vi "Drive Controller.vi"(8 "error in":errorcluster) -> ()   [LabVIEW 2018]
doc: "This VI executes continuously carrying out the current operation and responding to updates or new operation requests. It will often contain the timing or control code that is difficult to place directly in TeleOp. This VI generally opens all sensors and motors and isolates the rest of the robot code from knowing implementation details of how the operations are carried out."
uses:
  <vilib>/Rock Robotics/WPI/Framework/Completion Status.ctl
  2018 Practice Mecanum Command and Control/Drive/Implementation/Drive Setpoints.ctl
  2018 Practice Mecanum Command and Control/Drive/Implementation/Drive Operations.ctl
  <vilib>/Rock Robotics/WPI/SafetyOutput/WPI_SafetyOutputConfigMenu.ctl
  <vilib>/Rock Robotics/WPI/RobotDrive/WPI_RobotDriveOpen2MotorWithTalon.vi
panel:
  in  "Interactive Values":T1
  in  "Buttons":cluster{"Execute Cmd":bool, "Abort Cmd":bool}
  out "Command Timing":cluster{"Start Time (ms)":u32, "Iterations":i32}
  out "Status":T3
  out "Setpoints":T4(graph)
  out "Current\nCmd":string
  # "Tip: The graph shows the motor setpoints. It may also be helpful to observe inputs and sensor values.\nYou may also want to display tuning or debugging controls."
  # "Interactive Command: You may fill in the settings for a command\nand schedule it with the Execute button. You can observe and abort\nany command while fine tuning the code for the controller."
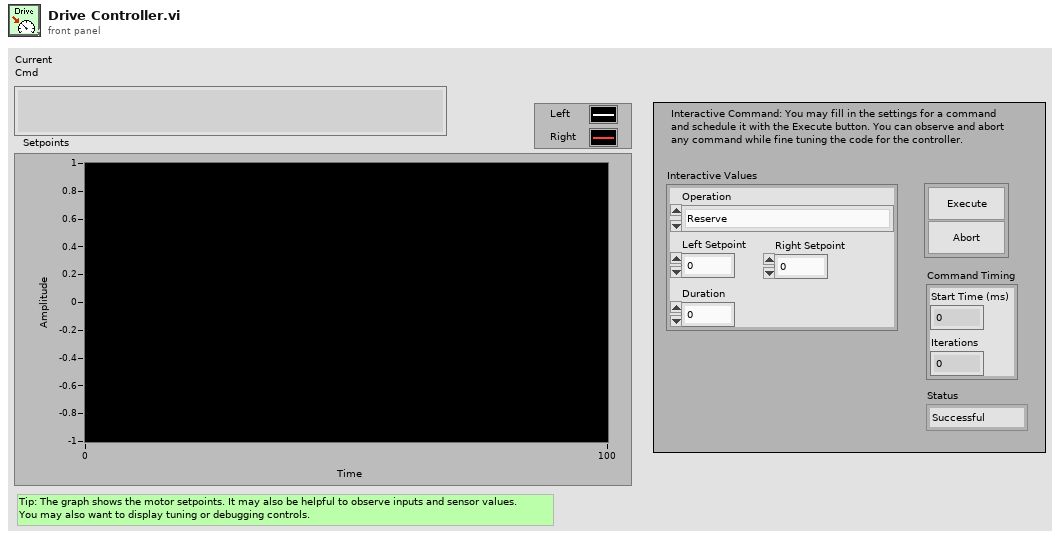
[diagram p1: front panel]
types:
  T1 = typedef "Drive Setpoints.ctl" = cluster{"Operation":T2, "Left Setpoint":dbl, "Right Setpoint":dbl, "Duration":dbl}
  T2 = typedef "Drive Operations.ctl" = enum16{"Reserve", "Read Current", "Immediate", "Drive for Time", "Drive for Distance"}
  T3 = typedef "Completion Status.ctl" = enum16{"Successful", "Aborted", "Incomplete"}
  T4 = cluster{"Left Setpoint":dbl, "Right Setpoint":dbl}
  T5 = typedef "WPI_SafetyOutputConfigMenu.ctl" = enum16{"Enable", "Disable"}
  T6 = typedef "WPI_RobotDriveDevRef.ctl" = cluster{"DevStatus":errorcluster, "Motors[]":T7[], "Square Inputs":bool, "Max Output":dbl}
  T7 = typedef "WPI_MotorControlDeviceRef.ctl" = cluster{"DeviceStatus":errorcluster, "Type":T8, "PWM":cluster{"PWM Channel":T9, "DeadBand":T10}, "CAN":cluster{"Device Number":u8, "SetOutput VI Ref":variant, "GetOutput VI Ref":variant, "Enable VI Ref":variant, "Disable VI Ref":variant, "Data":variant}, "Invert":bool, "DIO PWM":cluster{"PWM \"Enable\" Channel":T9, "DIOChannel":T11, "PWM Rate":dbl}}
  T8 = typedef "WPI_MotorControlType.ctl" = enum16{"PWM", "CAN", "DIO PWM"}
  T9 = typedef "FPGA_DIOPWMChannel.ctl" = enum8{"PWM 0", "PWM 1", "PWM 2", "PWM 3", "PWM 4", "PWM 5", "PWM 6", "PWM 7", "PWM 8", "PWM 9", "PWM MXP 0", "PWM MXP 1", "PWM MXP 2", "PWM MXP 3", "PWM MXP 4", "PWM MXP 5", "PWM MXP 6", "PWM MXP 7", "PWM MXP 8", "PWM MXP 9", "Invalid"}
  T10 = typedef "WPI_PWMDeadband.ctl" = cluster{"Name":string, "maxPositivePwm":i32, "minPositivePwm":i32, "centerPwm":i32, "maxNegativePwm":i32, "minNegativePwm":i32, "angularRange":u16}
  T11 = typedef "FPGA_DIOChannel.ctl" = enum8{"DIO 0", "DIO 1", "DIO 2", "DIO 3", "DIO 4", "DIO 5", "DIO 6", "DIO 7", "DIO 8", "DIO 9", "DIO MXP 0", "DIO MXP 1", "DIO MXP 2", "DIO MXP 3", "DIO MXP 4", "DIO MXP 5", "DIO MXP 6", "DIO MXP 7", "DIO MXP 8", "DIO MXP 9", "DIO MXP 10", "DIO MXP 11", "DIO MXP 12", "DIO MXP 13", "DIO MXP 14", "DIO MXP 15", "SPI Port CS1", "SPI Port CS2", "SPI Port CS3", "SPI Port MISO", "SPI Port MOSI", "Invalid"}
  T12 = typedef "Command Status Info.ctl" = cluster{"Name":string, "Status":T3, "notifier out":T13}
  T13 = typedef "Completion Notifier.ctl" = refnum<notifier>
  T14 = cluster{"SubSystem Data":T1, cluster{"Start Time (ms)":u32, "Iterations":i32}, cluster{"Command Info":T12, "Description":string, "Default Command":T1, "queue out":refnum<queue>, "Subsystem Name":string}}
  T15 = cluster{"SubSystem Data":T1, cluster{"Start Time (ms)":u32, "Iterations":i32}, "Default Command Arguments":cluster{"Command Info":T12, "Description":string, "Default Command":T1, "queue out":refnum<queue>, "Subsystem Name":string}}
  T16 = cluster{"Don't move motors while reserved":dbl, "Don't move motors while reserved":dbl}
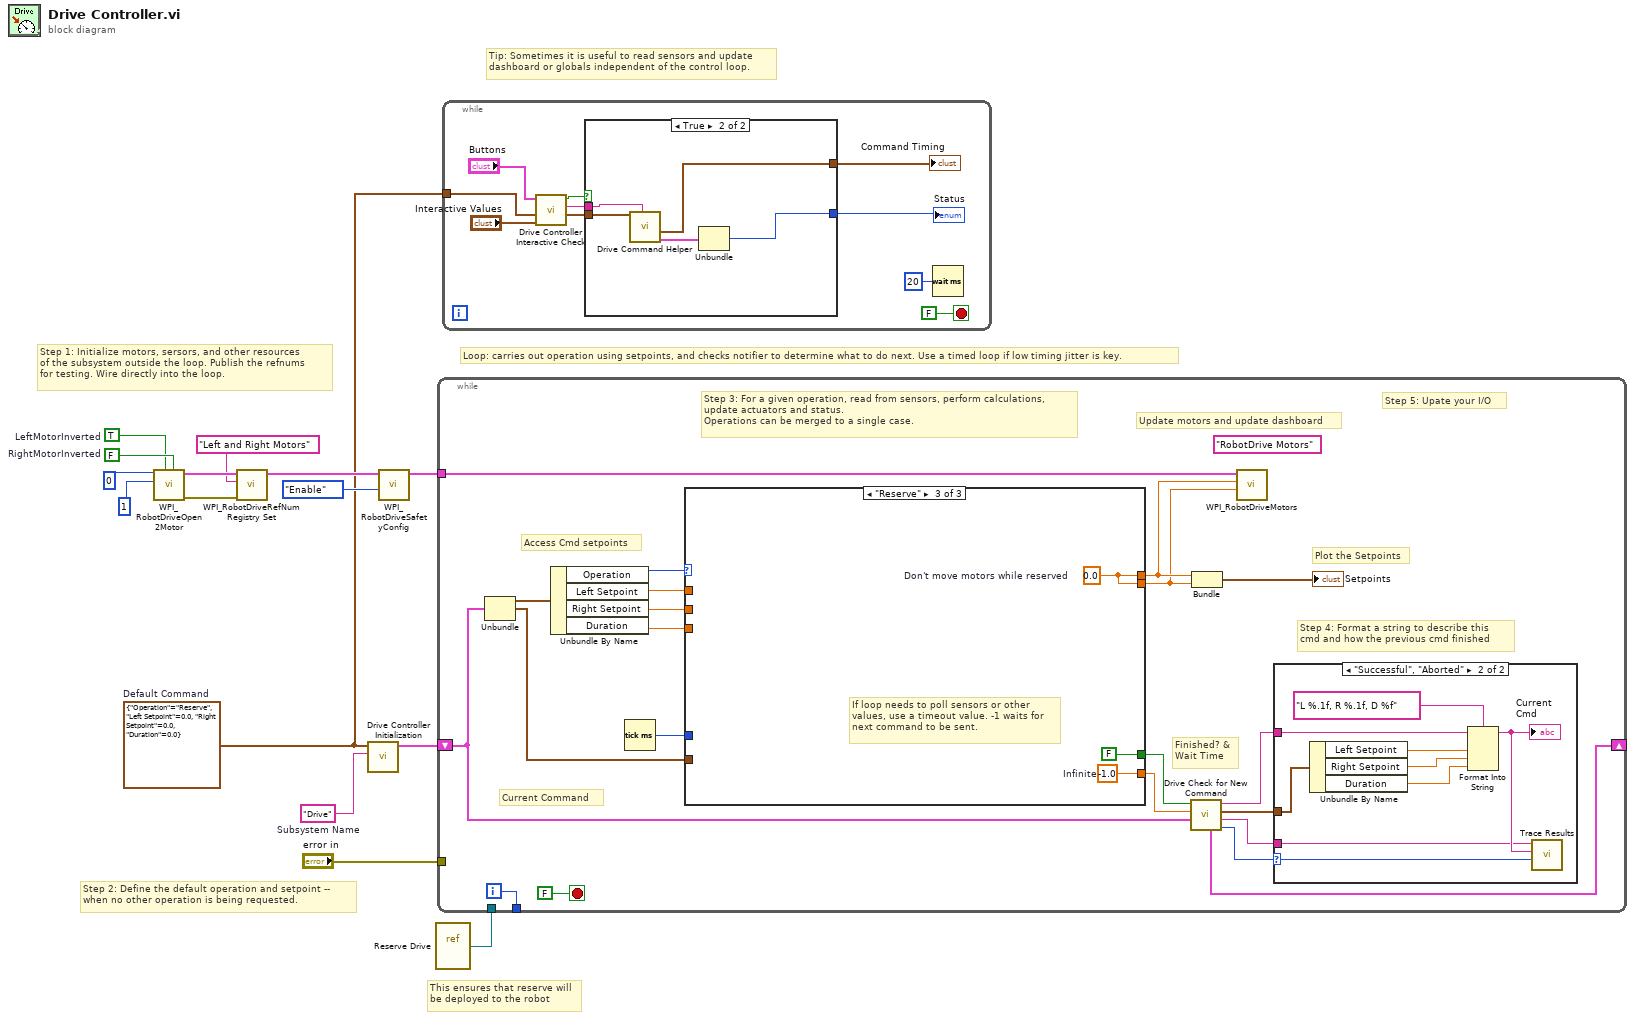
[diagram p0: block diagram]
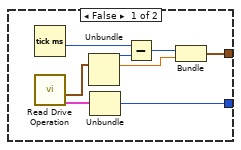
[diagram p2: hidden frame]
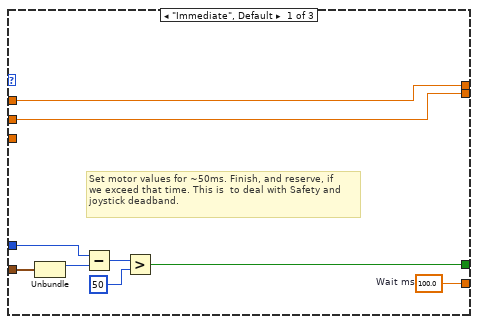
[diagram p4: hidden frame]
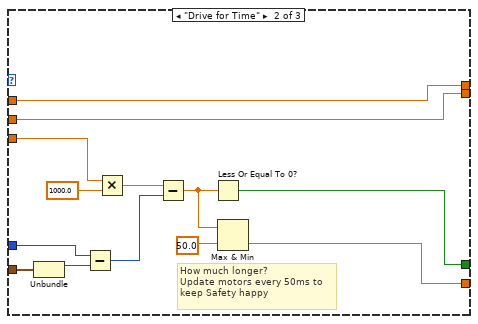
[diagram p5: hidden frame]
diagram:
  w11 = TRUE  # LeftMotorInverted
  w12 = FALSE  # RightMotorInverted
  w1 = T1 {"Operation"=enum."Reserve", "Left Setpoint"=0.0, "Right Setpoint"=0.0, "Duration"=0.0}  # Default Command
  w15 = "Drive"  # Subsystem Name
  # "This ensures that reserve will\nbe deployed to the robot"
  # "Tip: Sometimes it is useful to read sensors and update\ndashboard or globals independent of the control loop."
  # "Step 2: Define the default operation and setpoint --\nwhen no other operation is being requested."
  # "Step 1: Initialize motors, sersors, and other resources\nof the subsystem outside the loop. Publish the refnums\nfor testing. Wire directly into the loop."
  # "Loop: carries out operation using setpoints, and checks notifier to determine what to do next. Use a timed loop if low timing jitter is key."
  n1 = call-poly <vilib>:"WPI_RobotDriveOpen2Motor.vi"("Right Motor Inverted"=w12, "Left Motor Inverted"=w11, "Right Motor"=u8 1 ("Left Motor"), "Left Motor"=u8 0) -> ("error out"=w8:errorcluster, "RobotDriveDevRef"=w10:T6)  [unwired: 1 in, 5 out]
  n2 = call <vilib>:"WPI_RobotDriveRefNum Registry Set.vi"("error in (no error)"=w8, "refnum name"="Left and Right Motors", "RobotDriveDevRef"=w10) -> ("RobotDriveDevRef"=w7:T6)  [unwired: 1 in, 7 out]
  n3 = call "Drive Controller Initialization.vi"("Subsystem Name"=w15, "Default Command"=w1) -> ("Current Command"=w3:T14)  [unwired: 9 in]
  n4 = call <vilib>:"WPI_RobotDriveSafetyConfig.vi"("mode"=WPI_SafetyOutputConfigMenu."Enable", "RobotDriveDevRef"=w7) -> ("RobotDriveDevRef"=w5:T6)  [unwired: 8 in, 1 out]
  n5 = vi-ref "Reserve Drive.vi"() -> (w2:refnum<vi>)
  n6 = while {
    shift-right: [w23] -> _
    shift-left: w3 -> [w16]
    tunnel: [w35] -> _
    tunnel: w5 -> [w31]
    tunnel: "error in" -> [_]
    tunnel: w2 -> [_]
    i -> [w35]
    stop <- FALSE stop-if-true
    (unwired) "RobotDrive Motors" ("Name")
    # "Step 5: Upate your I/O"
    # "Step 4: Format a string to describe this\ncmd and how the previous cmd finished"
    # "Current Command"
    # "Update motors and update dashboard"
    # "Plot the Setpoints"
    # "Access Cmd setpoints"
    # "Finished? &\nWait Time"
    # "Step 3: For a given operation, read from sensors, perform calculations,\nupdate actuators and status.\nOperations can be merged to a single case."
    n7 = Unbundle(w16) -> ("SubSystem Data"=w30:T1, w17:cluster{"Start Time (ms)":u32, "Iterations":i32})  [unwired: 1 out]
    n8 = Unbundle By Name(w30) -> ("Operation"=w29:T2, "Left Setpoint"=w28:dbl, "Right Setpoint"=w27:dbl, "Duration"=w26:dbl)
    n9 = Tick Count (ms)() -> (millisecond timer value=w25:u32)
    n10 = case shown="\"Reserve\"" w29 {
      tunnel: [w54 w55 w70] -> w22
      tunnel: [w47 w62 FALSE ("ignore previous (F)")] -> w21
      tunnel: w17 -> [w46 w64 _]
      tunnel: [w53 w61 w68] -> w33
      tunnel: [w52 w60 w68] -> w32
      tunnel: w28 -> [w53 w61 _]
      tunnel: w27 -> [w52 w60 _]
      tunnel: w26 -> [_ w59 _]
      tunnel: w25 -> [w48 w58 _]
      frame "Immediate", Default {
        w54 = 100.0  # Wait ms
        # "Set motor values for ~50ms. Finish, and reserve, if\nwe exceed that time. This is  to deal with Safety and\njoystick deadband."
        n11 = Unbundle(w46) -> ("Start Time (ms)"=w49:u32)  [unwired: 1 out]
        n12 = Subtract(x=w48, y=w49) -> (x-y=w50:u32)
        n13 = Greater?(x=w50, y=u8 50 ("Left Motor")) -> (0:w47:bool)
      }
      frame "Drive for Time" {
        # "How much longer?\nUpdate motors every 50ms to\nkeep Safety happy"
        n14 = Unbundle(w64) -> ("Start Time (ms)"=w63:u32)  [unwired: 1 out]
        n15 = Subtract(x=w58, y=w63) -> (x-y=w67:u32)
        n16 = Multiply(x=w59, y=1000.0) -> (x*y=w66:dbl)
        n17 = Subtract(x=w66, y=w67) -> (x-y=w57:dbl)
        n18 = Less Or Equal To 0?(x=w57) -> (x <= 0?=w62:bool)
        n19 = Max & Min(x=w57, y=50.0) -> (min(x,y)=w55:dbl)  [unwired: 1 out]
      }
      frame "Reserve" {
        w68 = 0.0  # Don't move motors while reserved
        w70 = -1.0  # Infinite
        # "If loop needs to poll sensors or other\nvalues, use a timeout value. -1 waits for\nnext command to be sent."
      }
    }
    n20 = call "Drive Check for New Command.vi"("input cluster"=w16, "Wait time (ms)"=w22, "Finished?"=w21) -> ("Completion"=w24:T3, "Subsystem Name"=w18:string, "Current Command"=w19:T1, "Initial Trace String"=w20:string, "Next Command"=w23:T15)  [unwired: 4 in]
    n21 = Bundle("Don't move motors while reserved"=w33, "Don't move motors while reserved"=w32) -> (→"Setpoints":T16)  [unwired: 1 in]
    n22 = call <vilib>:"WPI_RobotDriveMotors.vi"("RightSpeed"=w32, "LeftSpeed"=w33, "RobotDriveDevRef"=w31) -> ()  [unwired: 1 in, 8 out]
    n23 = case shown="\"Successful\", \"Aborted\"" w24 {
      selector: w24 -> [_ w45]
      tunnel: w20 -> [_ w40]
      tunnel: w19 -> [_ w41]
      tunnel: w18 -> [_ w37]
      frame "Incomplete", Default {
        # "Continuing current command"
      }
      frame "Successful", "Aborted" {
        # "Report and setup for next command"
        n24 = Unbundle By Name(w41) -> ("Left Setpoint"=w43:dbl, "Right Setpoint"=w44:dbl, "Duration"=w38:dbl)
        n25 = Format Into String(format string="L %.1f, R %.1f, D %f", initial string=w40, w43, w44, w38) -> (resulting string=w39:string)  [unwired: 1 in, 1 out]
        "Current\nCmd" <- w39
        n26 = call <vilib>:"Trace Results.vi"("Status of previous command"=w45, "Description"=w39, "Subsystem"=w37) -> ()  [unwired: 9 in]
      }
    }
  }
  n27 = while {
    tunnel: w1 -> [w72]
    stop <- FALSE stop-if-true
    n28 = call "Drive Controller Interactive Check.vi"("Interactive Command In"="Interactive Values", "Default Command"=w72, "Buttons"="Buttons") -> ("Interactive Command Out"=w74:T1, "Trace String"=w75:string, "Schedule"=w76:bool)  [unwired: 6 in]
    n29 = case shown="True" w76 {
      tunnel: [w85 w93] -> w77
      tunnel: [w84 w89] -> w78
      tunnel: w75 -> [_ w91]
      tunnel: w74 -> [_ w90]
      frame False {
        n30 = Tick Count (ms)() -> (millisecond timer value=w88:u32)
        n31 = call "Read Drive Operation.vi"() -> ("Command Info"=w82:T12, "SubSystem Data"=w81:T1)  [unwired: 9 in, 1 out]
        n32 = Unbundle(w81) -> ("Operation"=w86:T2, "Left Setpoint"=w83:dbl)  [unwired: 2 out]
        n33 = Unbundle(w82) -> ("Status"=w85:T3)  [unwired: 2 out]
        n34 = Subtract(x=w88, y=w86) -> (x-y=w87:u32)
        n35 = Bundle(w87, "Left Setpoint"=w83) -> (w84:cluster{u32, "Left Setpoint":dbl})  [unwired: 1 in]
      }
      frame True {
        n36 = call "Drive Command Helper.vi"("Description"=w91, "SubSystem Data"=w90) -> ("Command Info Out"=w92:T12, "Command Timing"=w89:cluster{"Start Time (ms)":u32, "Iterations":i32})  [unwired: 7 in, 1 out]
        n37 = Unbundle(w92) -> ("Status"=w93:T3)  [unwired: 2 out]
      }
    }
    "Status" <- w77
    "Command Timing" <- w78
    n38 = Wait (ms)(milliseconds to wait=u32 20) -> ()  [unwired: 1 out]
  }
